vi "ADS1115_CONVERT_ONE_SAMPLE.vi"(0 "handle":u32, 5 "I2C Slave Address (0)":u8, 7 "Scale mV":u16=2, 11 "error in (no error)":errorcluster, 12 "options_i2c_write":T1, 13 "options_i2c_read":T1) -> (4 "handle out":u32, 6 "mV_out":u16, 8 "(hi.lo)":u16, 15 "error out":errorcluster)   [LabVIEW 2017]
uses:
  libMPSSE.lvlib
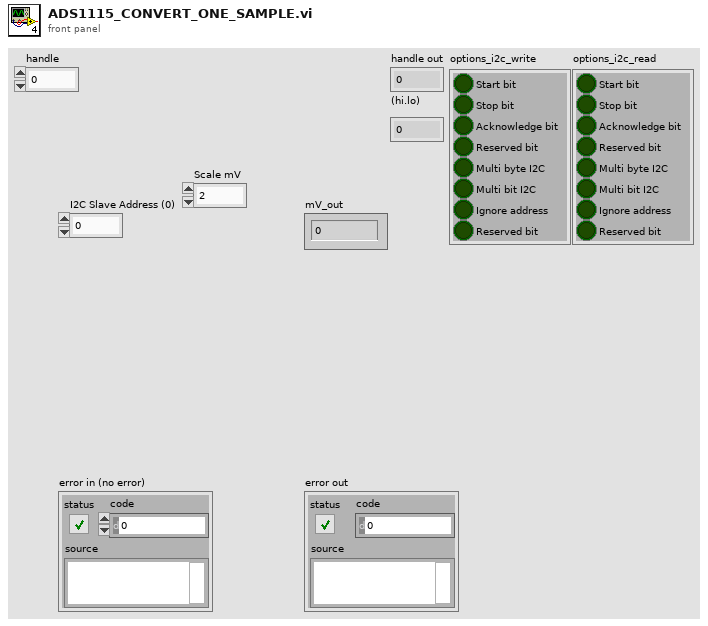
[diagram p1: front panel]
types:
  T1 = cluster{"Start bit":bool, "Stop bit":bool, "Acknowledge bit":bool, "Reserved bit":bool, "Multi byte I2C":bool, "Multi bit I2C":bool, "Ignore address":bool, "Reserved bit":bool}
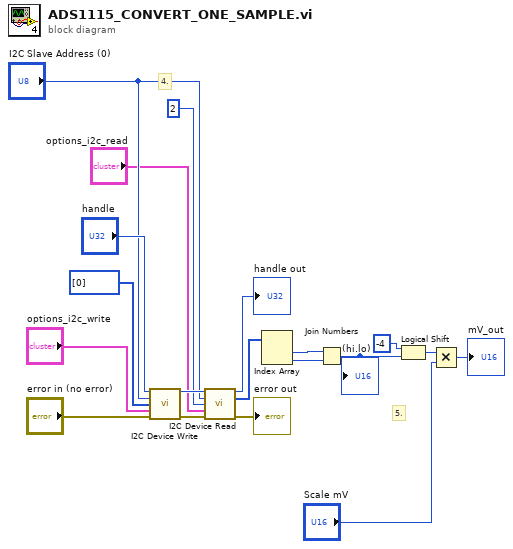
[diagram p0: block diagram]
diagram:
  # "5."
  # "4."
  n1 = call "I2C Device Write.vi"("handle"="handle", "deviceAddress"="I2C Slave Address (0)", "Data to write"=u8[] [0] ("Data"), "options"="options_i2c_write", "error in (no error)"="error in (no error)") -> ("handle out"=w9:u32, "error out"=w11:errorcluster)  [unwired: 8 in, 1 out]
  n2 = call "I2C Device Read.vi"("handle"=w9, "Slave device address"="I2C Slave Address (0)", "Size to transfer"=u8 2 ("Bytes To Read"), "options"="options_i2c_read", "error in (no error)"=w11) -> ("handle out"=→"handle out":u32, "Data read"=w1:u8[], "error out"=→"error out":errorcluster)  [unwired: 6 in, 2 out]
  n3 = Index Array(array=w1) -> (element #1=w15:u8, element #2=w16:u8)  [unwired: 2 in]
  n4 = Join Numbers(hi=w15, lo=w16) -> ((hi.lo)=w14:u16)
  "(hi.lo)" <- w14
  n5 = Logical Shift(y=i8 -4, x=w14) -> (x << y=w18:u16)
  n6 = Multiply(x=w18, y="Scale mV") -> (x*y=→"mV_out":u16)
